vi "SetClockRate.vi"(8 "error in (no error)":errorcluster, 10 "u32_I2Cclk":u32=100 caption="Clock Rate" min=100 max=4000 step=1 format="%d Kbps", 11 "I2COUSBSim in":refnum<class "I2COUSBSim.lvclass">) -> (0 "error out":errorcluster, 1 "Status":string, 3 "I2COUSBSim out":refnum<class "I2COUSBSim.lvclass">)   [LabVIEW 2020, in "I2COUSB.lvlib" / "I2COUSBSim.lvclass"]
doc: "Set the clock rate"
uses:
  I2COUSBSim.lvclass
  I2COUSBSim.lvclass/I2COUSBSim.ctl
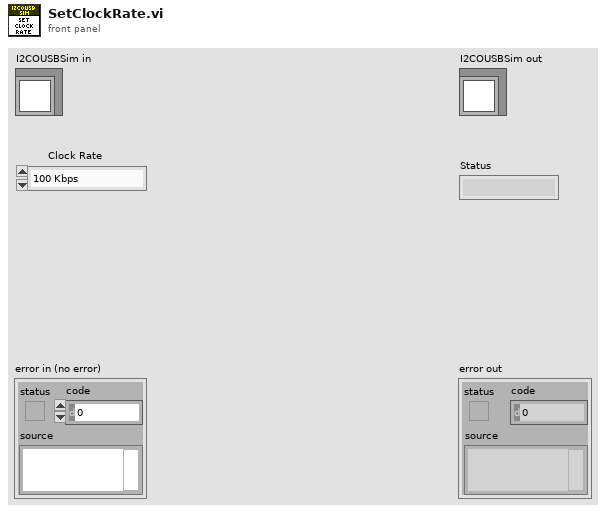
[diagram p1: front panel]
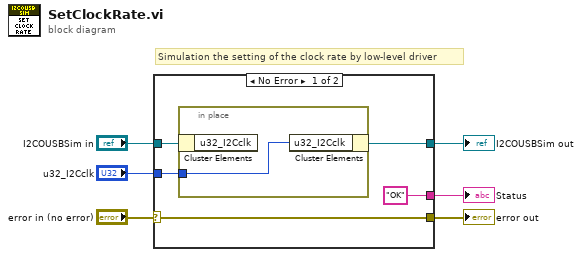
[diagram p0: block diagram]
diagram:
  # "Simulation the setting of the clock rate by low-level driver"
  n1 = case shown="No Error" "error in (no error)" {
    selector: "error in (no error)" -> [w11 w13]
    tunnel: "I2COUSBSim in" -> [w10 w14]
    tunnel: [w9 w14] -> w6
    tunnel: [w11 w13] -> w2
    tunnel: "u32_I2Cclk" -> [w8 _]
    tunnel: ["OK" ("Status") _] -> w1
    frame No Error {
      n2 = in-place {
        in-place-border: w8 -> [w12]
        n3 = in-place-cluster #1(w10) -> ()  [unwired: 1 out]
        n4 = in-place-cluster #1("u32_I2Cclk"=w12) -> (w9:refnum<class "I2COUSBSim.lvclass">)
      }
    }
    frame Error {
    }
  }
  "error out" <- w2
  "I2COUSBSim out" <- w6
  "Status" <- w1
